vi "FGV GE.vi"(6 "Enum":enum16{"lesen", "schreiben"}(ring), 11 "Ergebnis":sgl[](array[numeric])) -> (0 "Ergebnis %":sgl, 1 "Inter 3":sgl, 2 "Inter 2":sgl, 3 "Inter1":sgl, 5 "Ergebnis":sgl)   [LabVIEW 2020, in "EPA 1065.lvlib" / "HovaCAL Interference verificaton.lvlib"]
uses:
  HovaCAL Interference verificaton.lvlib
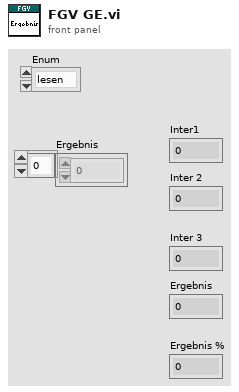
[diagram p1: front panel]
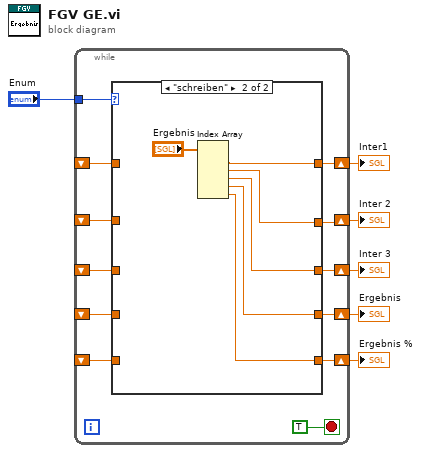
[diagram p0: block diagram]
diagram:
  n1 = while {
    shift-right: [w17] -> w6
    shift-left: _ -> [w14]
    shift-right: [w16] -> w5
    shift-left: _ -> [w13]
    shift-right: [w15] -> w4
    shift-left: _ -> [w12]
    tunnel: "Enum" -> [w11]
    shift-right: [w10] -> w2
    shift-left: _ -> [w8]
    shift-right: [w9] -> w1
    shift-left: _ -> [w7]
    stop <- TRUE stop-if-true
    n2 = case shown="\"schreiben\"" w11 {
      tunnel: [w23 w28] -> w17
      tunnel: [w22 w27] -> w16
      tunnel: [w21 w26] -> w15
      tunnel: w14 -> [w23 _]
      tunnel: w13 -> [w22 _]
      tunnel: w12 -> [w21 _]
      tunnel: [w20 w25] -> w10
      tunnel: [w19 w24] -> w9
      tunnel: w8 -> [w20 _]
      tunnel: w7 -> [w19 _]
      frame "lesen", Default {
      }
      frame "schreiben" {
        n3 = Index Array(array="Ergebnis") -> (element #1=w28:sgl, element #2=w27:sgl, element #3=w26:sgl, element #4=w25:sgl, element #5=w24:sgl)  [unwired: 5 in]
      }
    }
  }
  "Inter1" <- w6
  "Inter 2" <- w5
  "Inter 3" <- w4
  "Ergebnis" <- w2
  "Ergebnis %" <- w1
